vi "Format GPIO Data for Display.vi"(0 "gpio timestamps":T3[](array[typedef]), 5 "max samples to preallocate":i32=1000000, 7 "gpio to display":T1[](array[typedef])=[{"GPIO Bank"=enum."Ser0 GPIO Bank", "GPIO Number"=0}]) -> (4 "gpio timestamps waveform":digitalwaveform[](graph), 6 "error parsing timestamps":bool)   [LabVIEW 2023, in "GettingStarted_Common_148X_Host.lvlib"]
uses:
  GettingStarted_Common_148X_Host.lvlib
  <instrlib>/FlexRIO/CSI-2/v2/Host/Types/Host GPIO Bank Timestamp.ctl
  <instrlib>/FlexRIO/CSI-2/v2/FPGA/Types/Timestamp ID.ctl
  <instrlib>/FlexRIO/CSI-2/v2/FPGA/Types/GPIO Bank.ctl
  Types/GPIO Filter.ctl
  <instrlib>/FlexRIO/CSI-2/v2/Host/NI CSI-2 API Host v2.lvlib
  <instrlib>/FlexRIO/CSI-2/v2/FPGA/NI CSI-2 API FPGA v2.lvlib
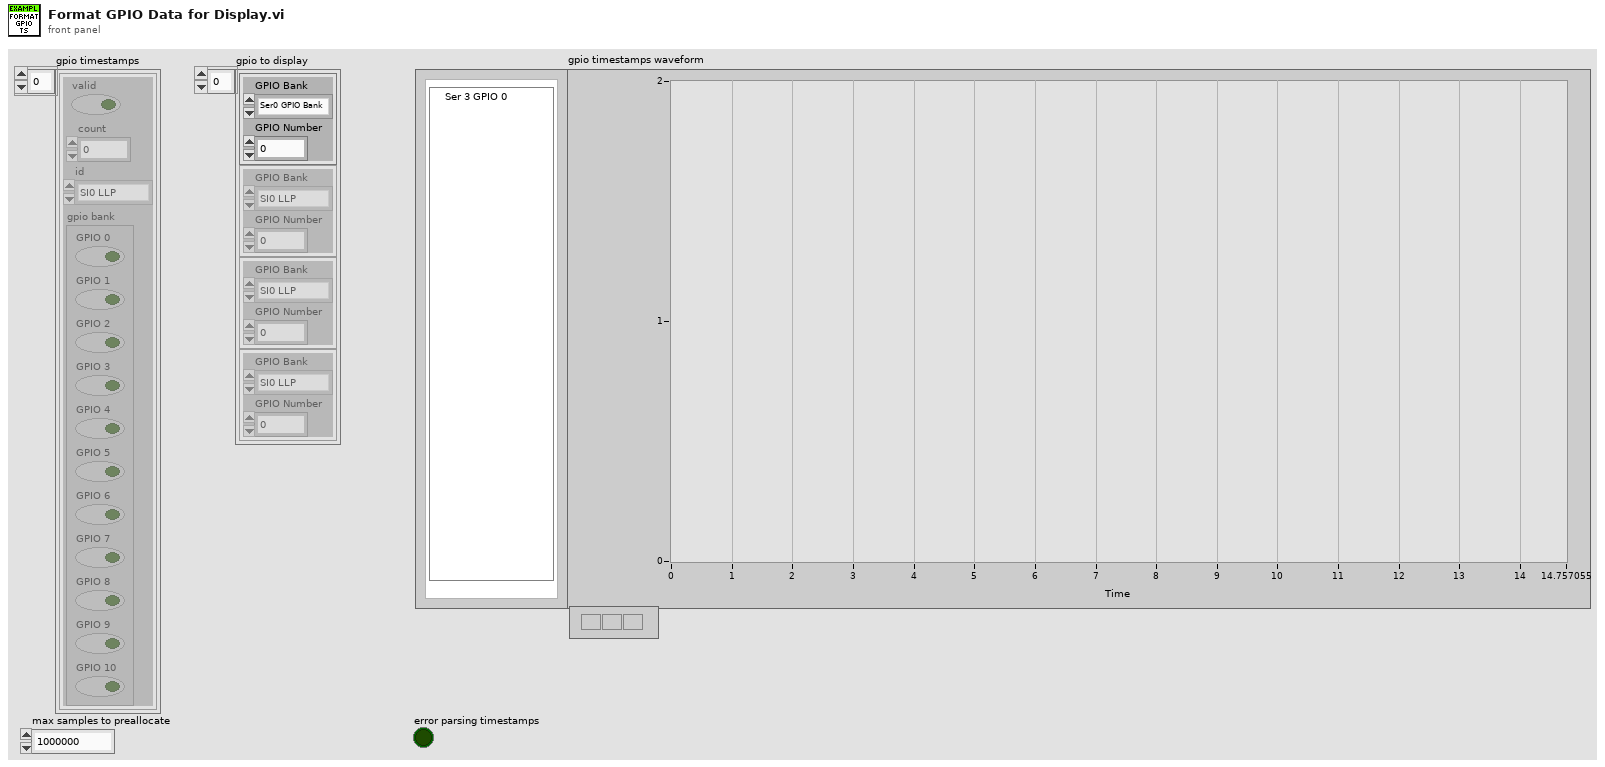
[diagram p1: front panel]
types:
  T1 = typedef "GettingStarted_Common_148X_Host.lvlib/GPIO Filter.ctl" = cluster{"GPIO Bank":T2, "GPIO Number":i32}
  T2 = typedef "NI CSI-2 API FPGA v2.lvlib/Timestamp ID.ctl" = enum8{"SI0 LLP", "SI1 LLP", "SI2 LLP", "SI3 LLP", "SI4 LLP", "SI5 LLP", "SI6 LLP", "SI7 LLP", "SO0 LLP", "SO1 LLP", "SO2 LLP", "SO3 LLP", "SO4 LLP", "SO5 LLP", "SO6 LLP", "SO7 LLP", "Ser0 GPIO Bank", "Ser1 GPIO Bank", "Ser2 GPIO Bank", "Ser3 GPIO Bank", "Ser4 GPIO Bank", "Ser5 GPIO Bank", "Ser6 GPIO Bank", "Ser7 GPIO Bank", "Des0 GPIO Bank", "Des1 GPIO Bank", "Des2 GPIO Bank", "Des3 GPIO Bank", "Des4 GPIO Bank", "Des5 GPIO Bank", "Des6 GPIO Bank", "Des7 GPIO Bank", "User0", "User1", "User2", "User3", "User4", "User5", "User6", "User7", "User8", "User9", "User10", "User11", "User12", "User13", "User14", "User15", "User16", "User17", "User18", "User19", "User20", "User21", "User22", "User23", "User24", "User25", "User26", "User27", "User28", "User29", "User30", "User31"}
  T3 = typedef "NI CSI-2 API Host v2.lvlib/Host GPIO Bank Timestamp.ctl" = cluster{"valid":bool, "count":u64, "id":T2, "gpio bank":T4}
  T4 = typedef "NI CSI-2 API FPGA v2.lvlib/GPIO Bank.ctl" = cluster{"GPIO 0":bool, "GPIO 1":bool, "GPIO 2":bool, "GPIO 3":bool, "GPIO 4":bool, "GPIO 5":bool, "GPIO 6":bool, "GPIO 7":bool, "GPIO 8":bool, "GPIO 9":bool, "GPIO 10":bool}
  T5 = cluster{"transitions":u64[], "t0":u64, "t0 valid":bool, "active index":i32, "GPIO data":cluster{cluster{u8[]}[]}}[]
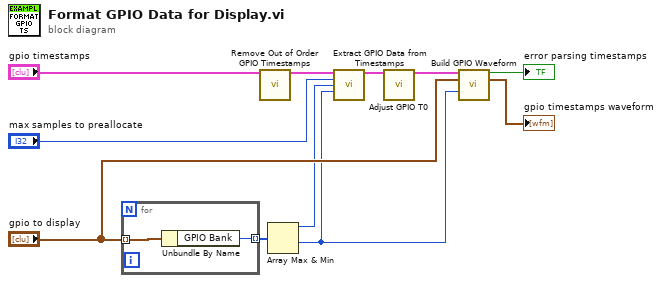
[diagram p0: block diagram]
diagram:
  n1 = for {
    tunnel: "gpio to display" -> [w13] mode=indexing
    tunnel: [w12] -> w8 mode=indexing
    n2 = Unbundle By Name(w13) -> ("GPIO Bank"=w12:T2)
  }
  n3 = call "Remove Out of Order GPIO Timestamps.vi"("gpio timestamps in"="gpio timestamps") -> ("gpio timestamps out"=w3:T3[])  [unwired: 13 in, 1 out]
  n4 = Array Max & Min(array=w8) -> (max value=w7:T2, min value=w5:T2)  [unwired: 2 out]
  n5 = call "Extract GPIO Data from Timestamps.vi"("gpio timestamps in"=w3, "max samples to preallocate"="max samples to preallocate", "max gpio bank"=w7, "min gpio bank"=w5) -> ("gpio timestamps out"=w2:T5)  [unwired: 11 in]
  n6 = call "Adjust GPIO T0.vi"("gpio timestamps in"=w2) -> ("gpio timestamps out"=w1:T5)  [unwired: 14 in]
  n7 = call "Build GPIO Waveform.vi"("gpio timestamps in"=w1, "gpio to display"="gpio to display", "min timestamp id"=w5) -> ("parsing error"=→"error parsing timestamps":bool, "waveform out"=→"gpio timestamps waveform":digitalwaveform[])  [unwired: 11 in]
